vi "Red Pitaya Control.vi"(8 "Error In":errorcluster, 10 "Server port":u16=1002, 11 "Server address":string="192.168.1.100") -> (0 "Error Out":errorcluster)   [LabVIEW 2015]
uses:
  File/Controls/File formats.ctl
panel:
  in  "Post-trigger points":i32
  in  "Trigger offset":i32
  in  "Read subset":bool
  out "Data File  Path":path
  in  "Auto-save file":bool=TRUE
  out "Trigger state":bool
  in  "Read trigger":bool=TRUE
  in  "FPGA Logic":enum16{"Digitizer", "Lock-in"}(ring)
  in  "Samples to record":u64=2097152 format="%x"
  in  "Trigger":bool
  in  "Read":bool
  in  "Arm":bool
  in  "Desimation rate":u64=125
  out "Temperature Chart":dbl(graph)=48.847186279148
  out "Thermometer":dbl(slide)=48.847186279148 scale=0.0..100.0
  in  "Read Temperature":bool=TRUE
  in  "Status offset":u64=8 format="%x"
  in  "Max Volts":dbl[](array[numeric])=[20.0, 1.0]
  out "x-y":u32=4294967295
  out "element":u32
  out "Phase  Graph":u32[](graph)
  in  "Mode":T1(ring)=enum."Digitizer test"
  out "Status response":u32=1
  in  "Status":bool
  out "Waveform Graph":dbl[][](graph)
  in  "Record":bool
  in  "Stop Server":bool
  out "bytes written":i32=8
  in  "Process Stop Button":bool
  out "Phase increment":u64=1717987
  in  "Output frequency":dbl=50000.0 format="%#_6p"
  in  "Samples to read":u64=67108864 format="%x"
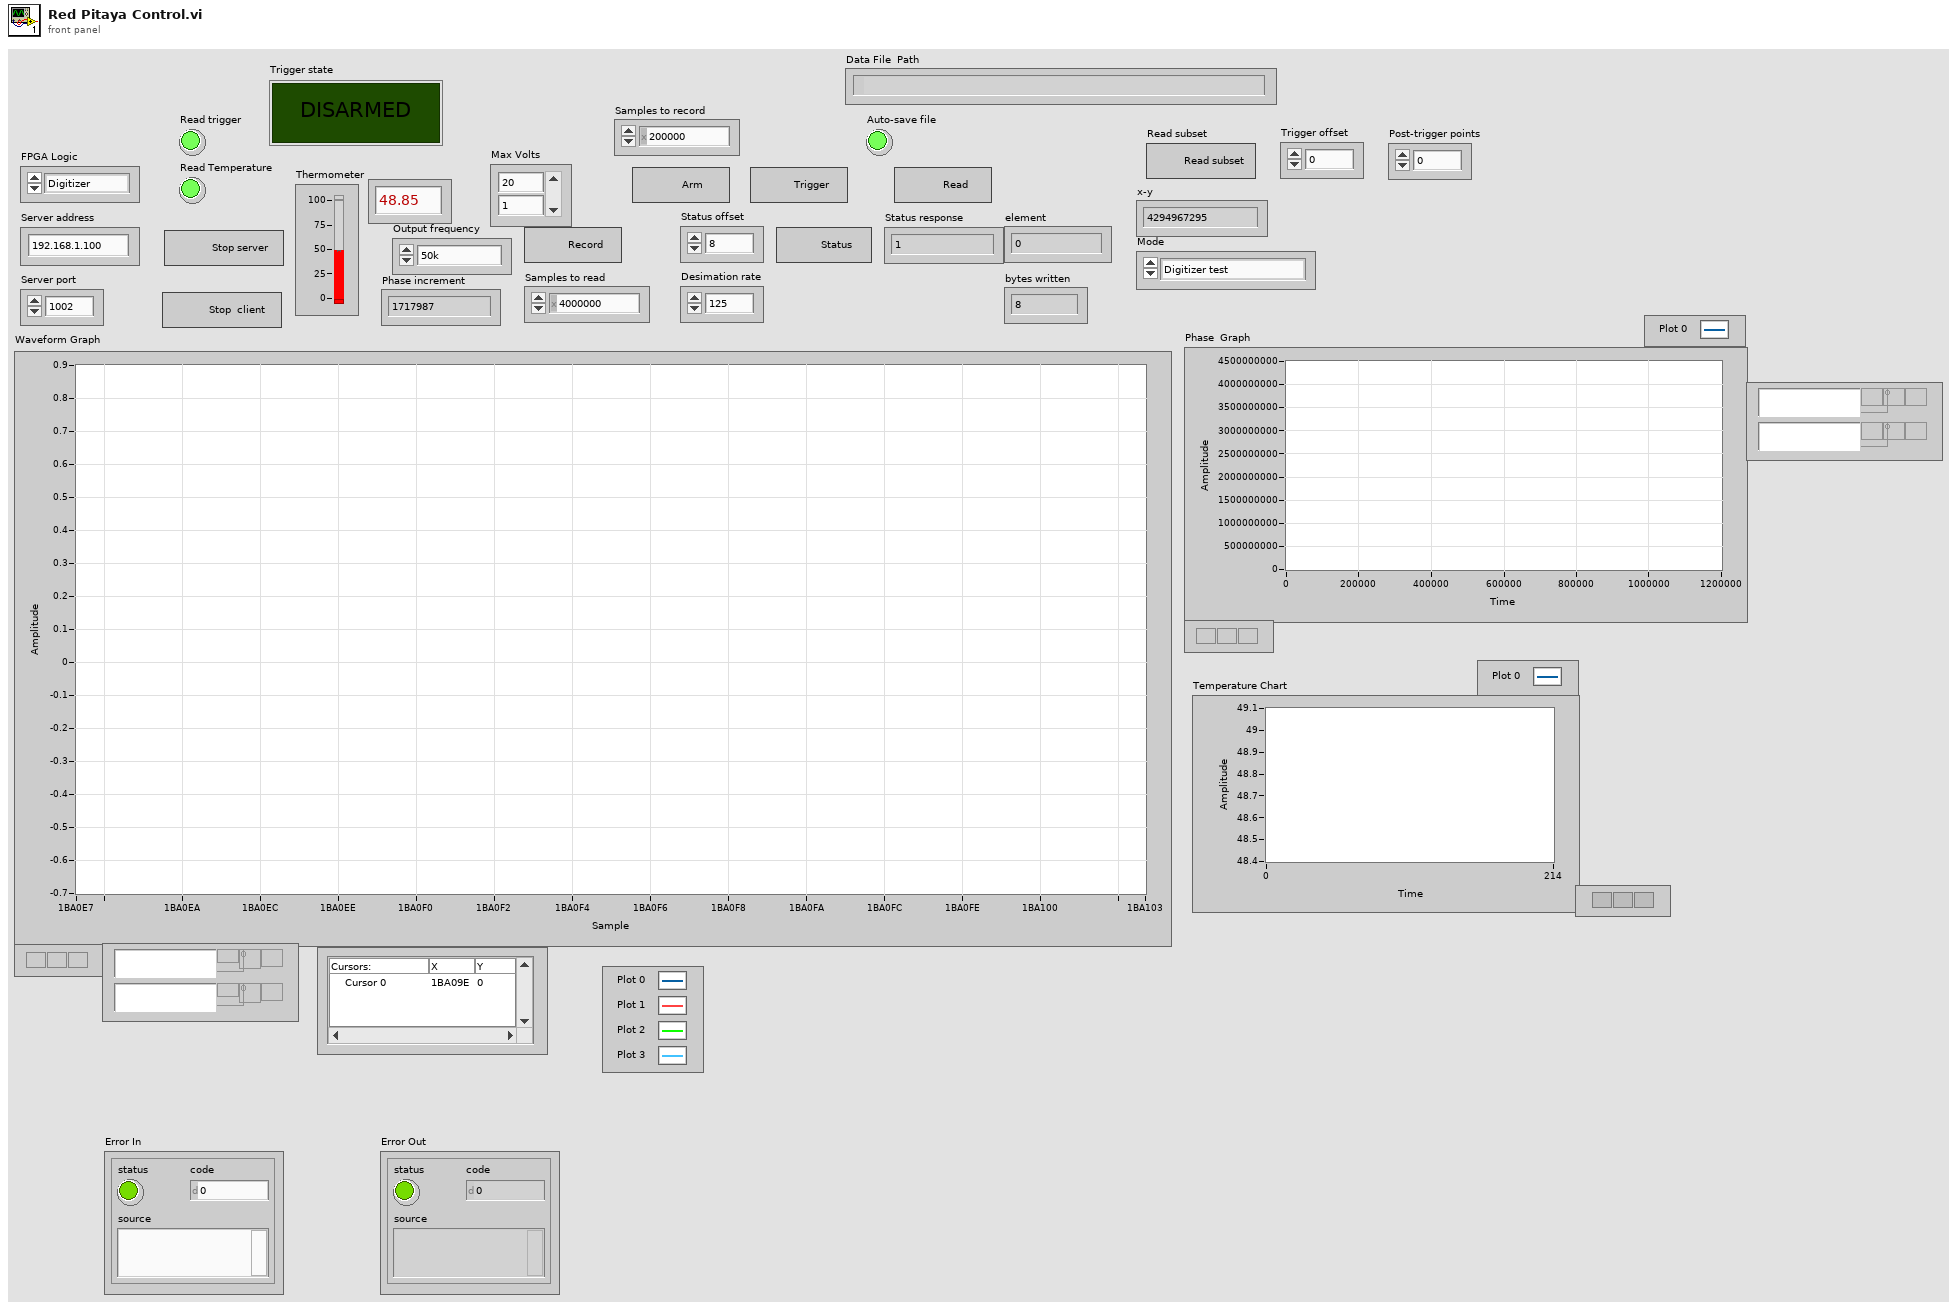
[diagram p1: front panel]
types:
  T1 = enum16{"Filter", "Lockin test", "Snapshot test", "Digitizer test"}
  T2 = enum16{"big-endian, network order", "native, host order", "little-endian"}
  T3 = typedef "File formats.ctl" = enum16{"TDMS", "ASCII", "BINARY"}
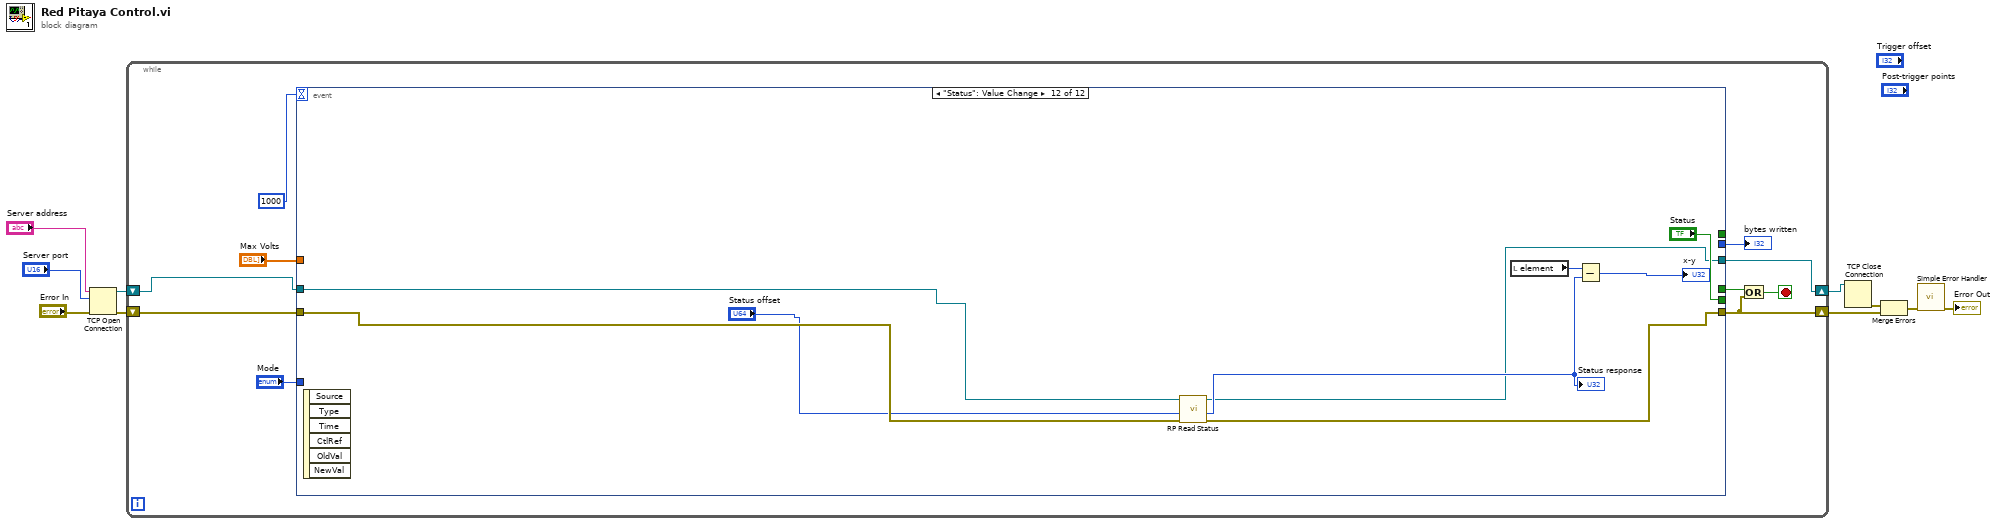
[diagram p0: block diagram]
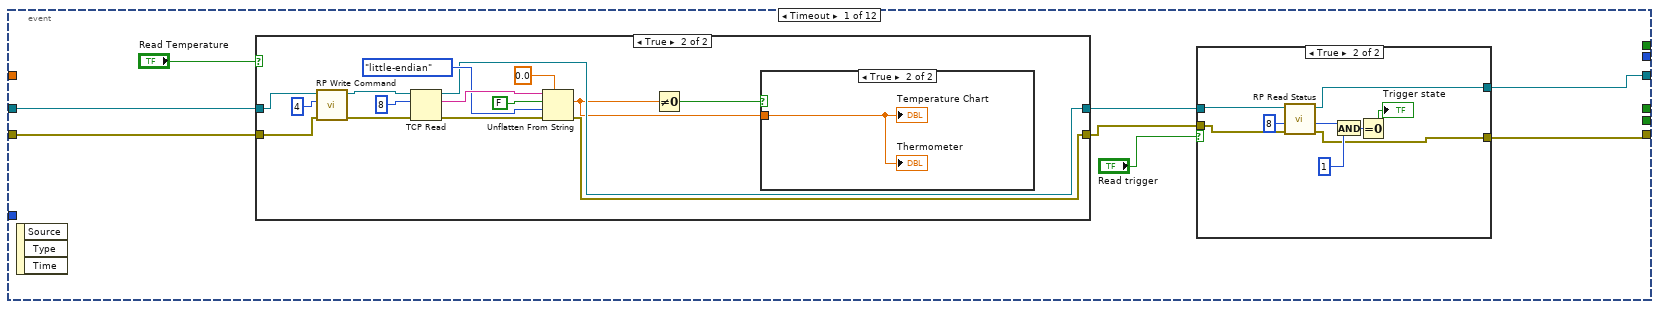
[diagram p2: hidden frame]
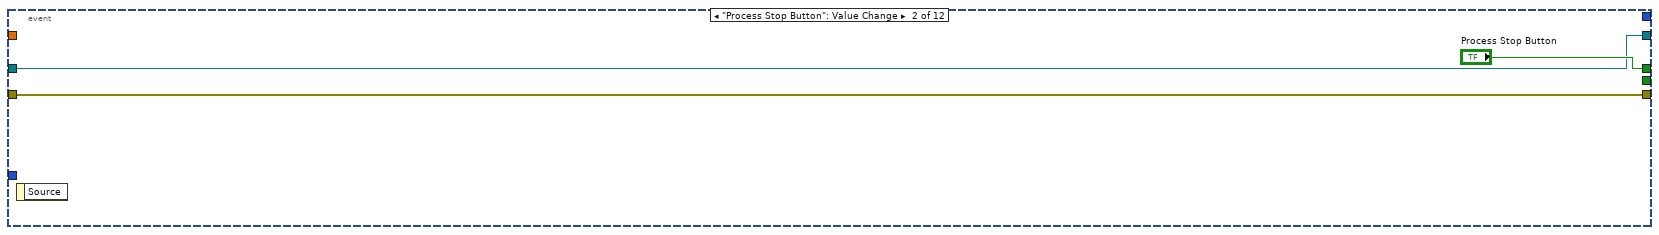
[diagram p6: hidden frame]
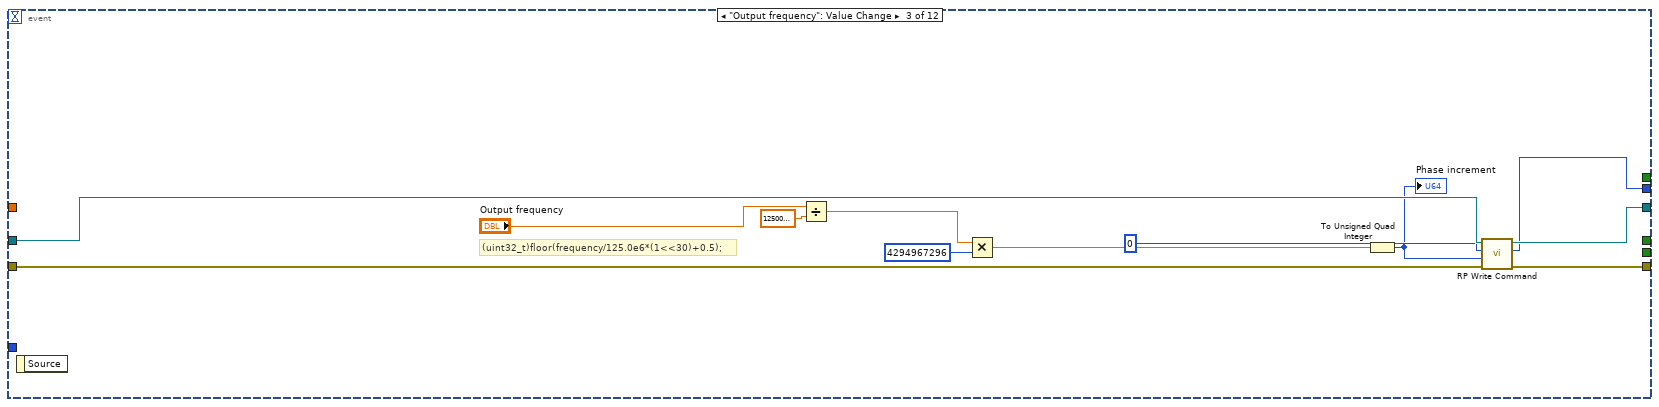
[diagram p7: hidden frame]
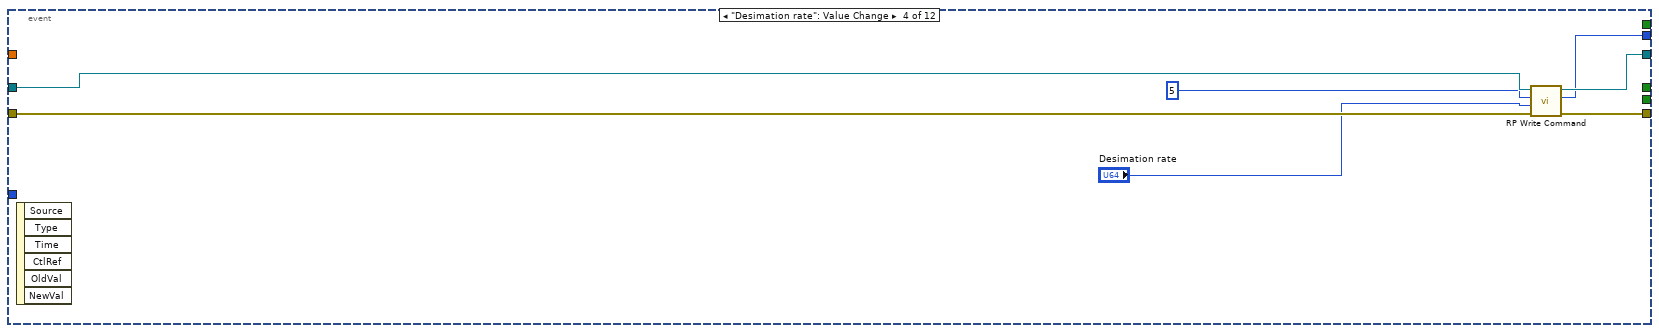
[diagram p8: hidden frame]
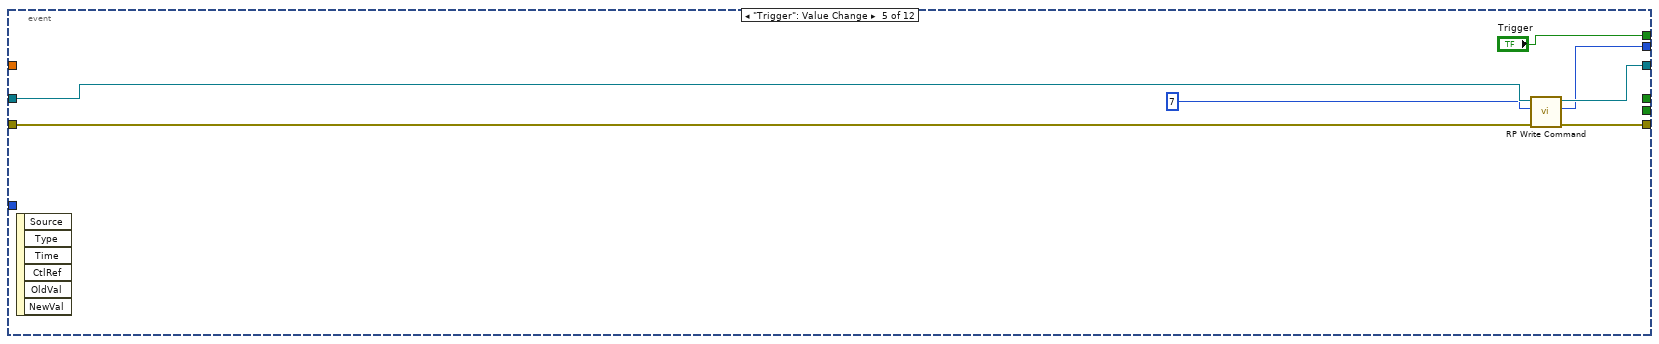
[diagram p9: hidden frame]
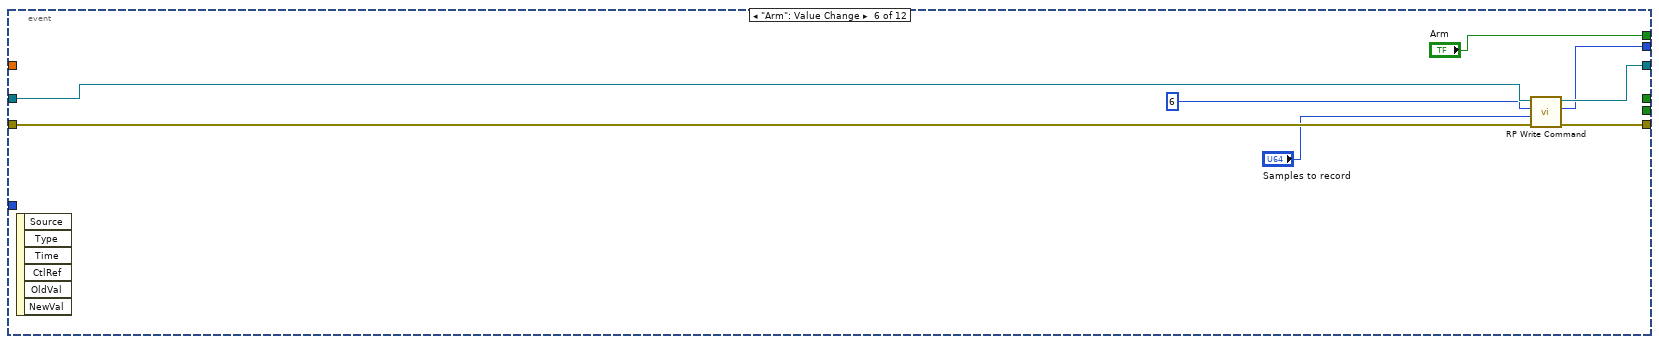
[diagram p10: hidden frame]
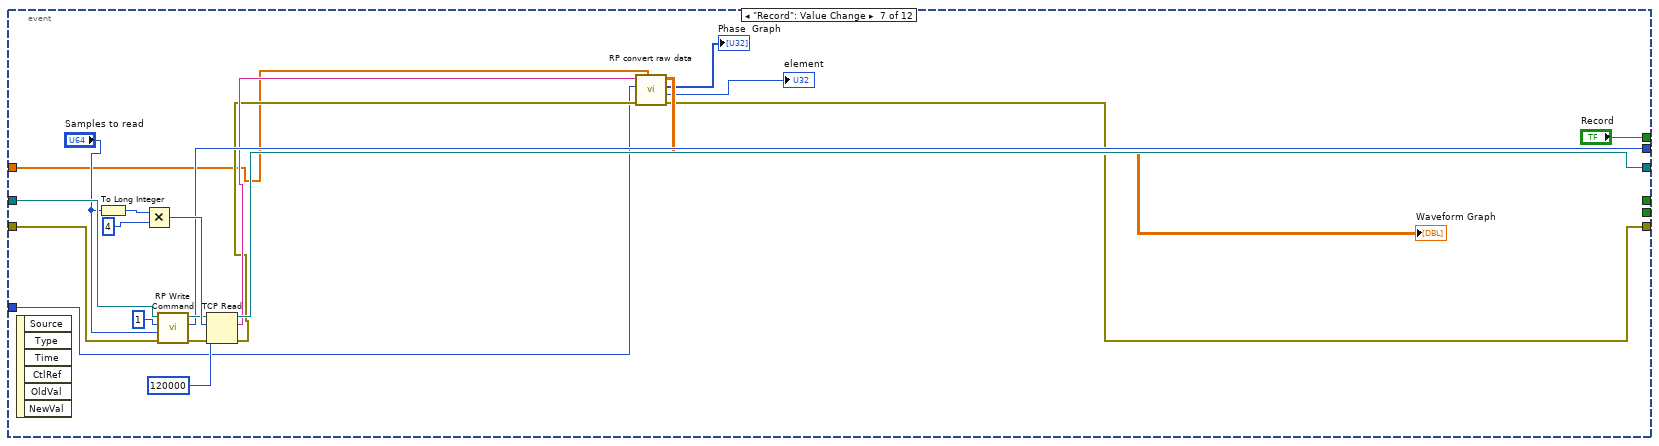
[diagram p11: hidden frame]
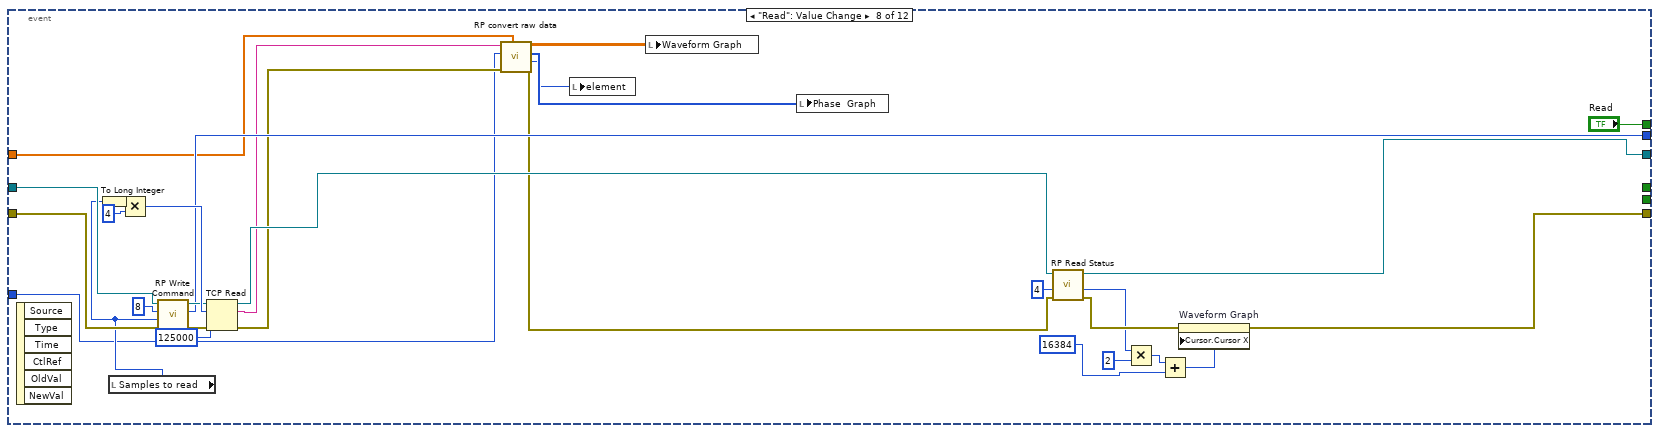
[diagram p12: hidden frame]
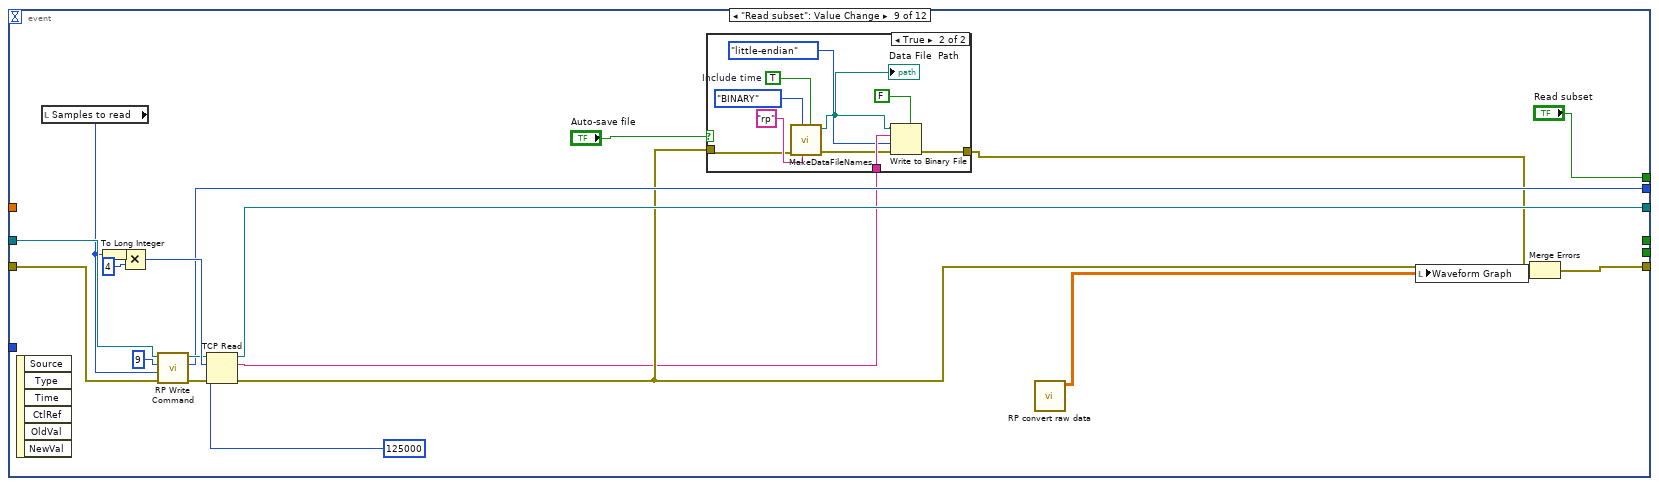
[diagram p13: hidden frame]
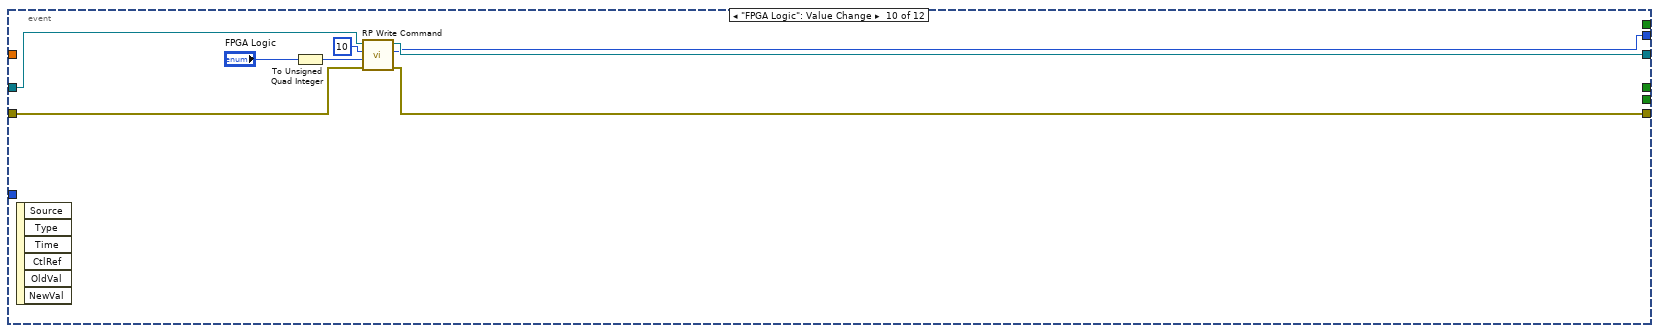
[diagram p15: hidden frame]
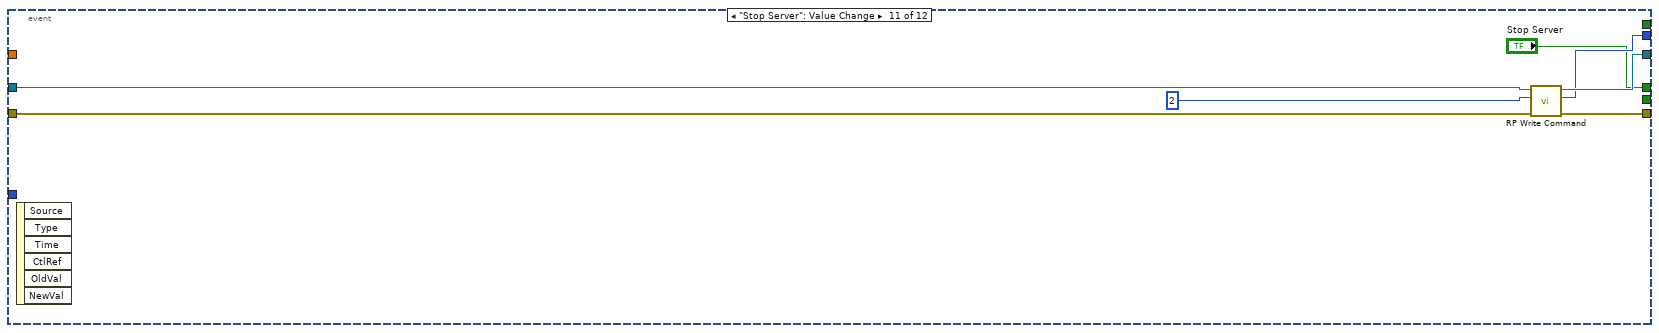
[diagram p16: hidden frame]
diagram:
  n1 = TCP Open Connection(address="Server address", remote port or service name="Server port", error in (no error)="Error In") -> (connection ID=w4:refnum<k5>, error out=w5:errorcluster)  [unwired: 2 in]
  n2 = while {
    shift-right: [w18] -> w3
    shift-left: w4 -> [w19]
    shift-right: [w16] -> w2
    shift-left: w5 -> [w20]
    stop <- w14 stop-if-true
    n3 = event shown="[11] \"Status\": Value Change" {
      selector: _ -> [_ _ _ _ _ _ _ _ _ _ _ _]
      dyn-events: _ -> [_ _ _ _ _ _ _ _ _ _ _ _]
      timeout: 1000 -> [_ _ _ _ _ _ _ _ _ _ _ _]
      tunnel: w20 -> [w26 w59 w67 w79 w86 w94 w108 w140 w159 w183 w190 w196]
      tunnel: w19 -> [w27 w58 w66 w78 w85 w93 w111 w143 w162 w182 w188 w192]
      tunnel: [w22 w59 w62 w75 w82 w90 w99 w137 w149 w178 w187 w195] -> w16
      tunnel: [w21 w58 w63 w76 w83 w91 w113 w133 w155 w177 w186 w193] -> w18
      tunnel: [_ "Process Stop Button" _ _ _ _ _ _ _ _ "Stop Server" _] -> w15
      tunnel: [_ _ _ _ _ _ _ _ _ _ _ "Status"] -> _
      tunnel: [_ _ w61 w74 w81 w89 w106 w138 w157 w176 w185 _] -> w17
      tunnel: [_ _ _ _ "Trigger" "Arm" "Record" "Read" "Read subset" _ _ _] -> _
      tunnel: "Max Volts" -> [_ _ _ _ _ _ w95 w130 _ _ _ _]
      tunnel: "Mode" -> [_ _ _ _ _ _ w96 w116 _ _ _ _]
      event Timeout {
        n4 = event-data() -> ()  [unwired: 1 in, 3 out]
        n5 = case shown="True" "Read Temperature" {
          tunnel: w27 -> [w41 w56]
          tunnel: w26 -> [w40 w55]
          tunnel: [w41 w44] -> w24
          tunnel: [w40 w46] -> w23
          frame False {
          }
          frame True {
            n6 = call "RP Write Command.vi"("Error In"=w55, "Command number"=u64 4, "connection ID"=w56) -> ("Error Out"=w47:errorcluster, "connection ID out"=w45:refnum<k5>)  [unwired: 6 in, 1 out]
            n7 = TCP Read(connection ID=w45, bytes to read=8, error in (no error)=w47) -> (connection ID out=w44:refnum<k5>, data out=w53:string, error out=w51:errorcluster)  [unwired: 2 in]
            n8 = Unflatten From String(type=0.0, binary string=w53, data includes array or string size? (T)=FALSE, byte order (0:big-endian, network order)=T2."little-endian", error in (no error)=w51) -> (value=w43:dbl, error out=w46:errorcluster)  [unwired: 1 out]
            n9 = Not Equal To 0?(x=w43) -> (x != 0?=w42:bool)
            n10 = case shown="True" w42 {
              tunnel: w43 -> [_ w57]
              frame False {
              }
              frame True {
                "Thermometer" <- w57
                "Temperature Chart" <- w57
              }
            }
          }
        }
        n11 = case shown="True" "Read trigger" {
          tunnel: w24 -> [w29 w38]
          tunnel: w23 -> [w30 w39]
          tunnel: [w30 w34] -> w22
          tunnel: [w29 w31] -> w21
          frame False {
          }
          frame True {
            n12 = call "RP Read Status.vi"("Error In"=w39, "Status offset"=u64 8, "connection ID"=w38) -> ("Error Out"=w34:errorcluster, "Status response"=w36:u32, "connection ID out"=w31:refnum<k5>)  [unwired: 6 in]
            n13 = And(x=w36, y=u32 1) -> (x .and. y?=w33:u32)
            n14 = Equal To 0?(x=w33) -> (x = 0?=→"Trigger state":bool)
          }
        }
      }
      event "Process Stop Button": Value Change {
        n15 = event-data() -> ()  [unwired: 1 in, 1 out]
      }
      event "Output frequency": Value Change {
        # "(uint32_t)floor(frequency/125.0e6*(1<<30)+0.5);"
        n16 = event-data() -> ()  [unwired: 1 in, 1 out]
        n17 = Divide(x="Output frequency", y=125000000.0) -> (x/y=w69:dbl)
        n18 = Multiply(x=w69, y=i64 4294967296) -> (x*y=w68:dbl)
        n19 = To Unsigned Quad Integer(1:w68) -> (0:w64:u64)
        "Phase increment" <- w64
        n20 = call "RP Write Command.vi"("Error In"=w67, "Command payload"=w64, "Command number"=u64 0, "connection ID"=w66) -> ("Error Out"=w62:errorcluster, "bytes written"=w61:i32, "connection ID out"=w63:refnum<k5>)  [unwired: 5 in]
      }
      event "Desimation rate": Value Change {
        n21 = event-data() -> ()  [unwired: 1 in, 6 out]
        n22 = call "RP Write Command.vi"("Error In"=w79, "Command payload"="Desimation rate", "Command number"=u64 5, "connection ID"=w78) -> ("Error Out"=w75:errorcluster, "bytes written"=w74:i32, "connection ID out"=w76:refnum<k5>)  [unwired: 5 in]
      }
      event "Trigger": Value Change {
        n23 = event-data() -> ()  [unwired: 1 in, 6 out]
        n24 = call "RP Write Command.vi"("Error In"=w86, "Command number"=u64 7, "connection ID"=w85) -> ("Error Out"=w82:errorcluster, "bytes written"=w81:i32, "connection ID out"=w83:refnum<k5>)  [unwired: 6 in]
      }
      event "Arm": Value Change {
        n25 = event-data() -> ()  [unwired: 1 in, 6 out]
        n26 = call "RP Write Command.vi"("Error In"=w94, "Command payload"="Samples to record", "Command number"=u64 6, "connection ID"=w93) -> ("Error Out"=w90:errorcluster, "bytes written"=w89:i32, "connection ID out"=w91:refnum<k5>)  [unwired: 5 in]
      }
      event "Record": Value Change {
        n27 = event-data() -> ()  [unwired: 1 in, 6 out]
        n28 = To Long Integer(number="Samples to read") -> (32bit integer=w105:i32)
        n29 = Multiply(x=w105, y=4) -> (x*y=w112:i32)
        n30 = call "RP Write Command.vi"("Error In"=w108, "Command payload"="Samples to read", "Command number"=u64 1, "connection ID"=w111) -> ("Error Out"=w107:errorcluster, "bytes written"=w106:i32, "connection ID out"=w109:refnum<k5>)  [unwired: 5 in]
        n31 = TCP Read(connection ID=w109, bytes to read=w112, error in (no error)=w107, 9:120000 ("timeout ms (25000)")) -> (connection ID out=w113:refnum<k5>, data out=w102:string, error out=w100:errorcluster)  [unwired: 1 in]
        n32 = call "RP convert raw data.vi"("Max Volts"=w95, "Error In"=w100, "Format"=w96, "data stream"=w102) -> ("Error Out"=w99:errorcluster, "element"=→"element":u32, "phase out"=→"Phase  Graph":u32[], "data out"=→"Waveform Graph":dbl[][])  [unwired: 4 in]
      }
      event "Read": Value Change {
        n33 = event-data() -> ()  [unwired: 1 in, 6 out]
        n34 = local read "Samples to read"() -> (w132:u64)
        n35 = To Long Integer(number=w132) -> (32bit integer=w135:i32)
        n36 = Multiply(x=w135, y=4) -> (x*y=w144:i32)
        n37 = call "RP Write Command.vi"("Error In"=w140, "Command payload"=w132, "Command number"=u64 8, "connection ID"=w143) -> ("Error Out"=w139:errorcluster, "bytes written"=w138:i32, "connection ID out"=w141:refnum<k5>)  [unwired: 5 in]
        n38 = TCP Read(connection ID=w141, bytes to read=w144, error in (no error)=w139, 9:125000 ("timeout ms (25000)")) -> (connection ID out=w134:refnum<k5>, data out=w129:string, error out=w118:errorcluster)  [unwired: 1 in]
        n39 = call "RP convert raw data.vi"("Max Volts"=w130, "Error In"=w118, "Format"=w116, "data stream"=w129) -> ("Error Out"=w117:errorcluster, "element"=w126:u32, "phase out"=w127:u32[], "data out"=w128:dbl[][])  [unwired: 4 in]
        n40 = local write "element"(w126) -> ()
        n41 = local write "Waveform Graph"(w128) -> ()
        n42 = local write "Phase  Graph"(w127) -> ()
        n43 = call "RP Read Status.vi"("Error In"=w117, "Status offset"=u64 4, "connection ID"=w134) -> ("Error Out"=w124:errorcluster, "Status response"=w123:u32, "connection ID out"=w133:refnum<k5>)  [unwired: 6 in]
        n44 = Multiply(x=w123, y=u32 2) -> (x*y=w121:u32)
        n45 = Add(x=w121, y=16384) -> (x+y=w119:u32)
        n46 = property on="Waveform Graph" class="WFGraph (strict)"(error in=w124, "Cursor.Cursor X"=w119) -> (error out=w137:errorcluster)  [unwired: 1 in, 1 out]
      }
      event "Read subset": Value Change {
        n47 = event-data() -> ()  [unwired: 1 in, 6 out]
        n48 = local read "Samples to read"() -> (w154:u64)
        n49 = To Long Integer(number=w154) -> (32bit integer=w156:i32)
        n50 = Multiply(x=w156, y=4) -> (x*y=w163:i32)
        n51 = call "RP Write Command.vi"("Error In"=w159, "Command payload"=w154, "Command number"=u64 9, "connection ID"=w162) -> ("Error Out"=w158:errorcluster, "bytes written"=w157:i32, "connection ID out"=w160:refnum<k5>)  [unwired: 5 in]
        n52 = TCP Read(connection ID=w160, bytes to read=w163, error in (no error)=w158, 9:125000 ("timeout ms (25000)")) -> (connection ID out=w155:refnum<k5>, data out=w147:string, error out=w150:errorcluster)  [unwired: 1 in]
        n53 = case shown="True" "Auto-save file" {
          tunnel: w150 -> [w165 w174]
          tunnel: w147 -> [_ w171]
          tunnel: [w165 w166] -> w148
          frame False {
          }
          frame True {
            w172 = TRUE  # Include time
            n54 = call "MakeDataFileNames.vi"("Include time"=w172, "File Prefix"="rp", "File format"=File_formats."BINARY", "Error In"=w174) -> ("Error Out"=w168:errorcluster, "Data File  Path"=w169:path)  [unwired: 5 in, 1 out]
            "Data File  Path" <- w169
            n55 = Write to Binary File(file (use dialog)=w169, data=w171, error in=w168, 5:FALSE ("prepend array or string size? (T)"), 9:T2."little-endian" ("byte order (0:big-endian, network order)")) -> (error out=w166:errorcluster)  [unwired: 1 in, 2 out]
          }
        }
        n56 = call "RP convert raw data.vi"() -> ("data out"=w146:dbl[][])  [unwired: 8 in, 3 out]
        n57 = local write "Waveform Graph"(w146) -> ()
        n58 = Merge Errors(w150, w148) -> (w149:errorcluster)
      }
      event "FPGA Logic": Value Change {
        n59 = event-data() -> ()  [unwired: 1 in, 6 out]
        n60 = To Unsigned Quad Integer(1:"FPGA Logic") -> (0:w180:u64)
        n61 = call "RP Write Command.vi"("Error In"=w183, "Command payload"=w180, "Command number"=u64 10, "connection ID"=w182) -> ("Error Out"=w178:errorcluster, "bytes written"=w176:i32, "connection ID out"=w177:refnum<k5>)  [unwired: 5 in]
      }
      event "Stop Server": Value Change {
        n62 = event-data() -> ()  [unwired: 1 in, 6 out]
        n63 = call "RP Write Command.vi"("Error In"=w190, "Command number"=u64 2, "connection ID"=w188) -> ("Error Out"=w187:errorcluster, "bytes written"=w185:i32, "connection ID out"=w186:refnum<k5>)  [unwired: 6 in]
      }
      event "Status": Value Change {
        n64 = event-data() -> ()  [unwired: 1 in, 6 out]
        n65 = call "RP Read Status.vi"("Error In"=w196, "Status offset"="Status offset", "connection ID"=w192) -> ("Error Out"=w195:errorcluster, "Status response"=w194:u32, "connection ID out"=w193:refnum<k5>)  [unwired: 6 in]
        "Status response" <- w194
        n66 = local read "element"() -> (w198:u32)
        n67 = Subtract(x=w198, y=w194) -> (x-y=→"x-y":u32)
      }
    }
    "bytes written" <- w17
    n68 = Or(x=w15, y=w16) -> (x .or. y?=w14:bool)
  }
  n69 = TCP Close Connection(connection ID=w3) -> (error out=w7:errorcluster)  [unwired: 2 in, 1 out]
  n70 = Merge Errors(w7, w2) -> (w6:errorcluster)
  n71 = call <vilib>:"Simple Error Handler.vi"("error in (no error)"=w6) -> ("error out"=→"Error Out":errorcluster)  [unwired: 4 in, 4 out]
